vi "Write Message.vi"(10 "Message":string, 11 "LogMessage In":refnum<class "AbstractLogMessage.lvclass">) -> (3 "LogMessage Out":refnum<class "AbstractLogMessage.lvclass">)   [LabVIEW 2020, in "AbstractLogMessage.lvclass"]
uses:
  AbstractLogMessage.lvclass
  AbstractLogMessage.lvclass/AbstractLogMessage.ctl
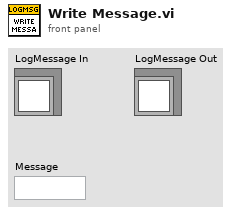
[diagram p1: front panel]
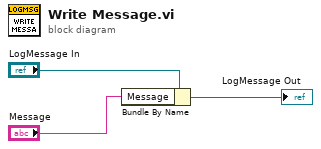
[diagram p0: block diagram]
diagram:
  n1 = Bundle By Name(cluster="LogMessage In", "Message"="Message") -> (→"LogMessage Out":refnum<class "AbstractLogMessage.lvclass">)
